vi "chr63204A_Mode_selector_Lowlevel.vi"(8 "error in (no error)":errorcluster, 10 "Mode":T1(ring), 11 "VISA resource name":refnum<visa-resource-name>) -> (0 "error out":errorcluster, 3 "VISA resource name out":refnum<visa-resource-name>)   [LabVIEW 2020]
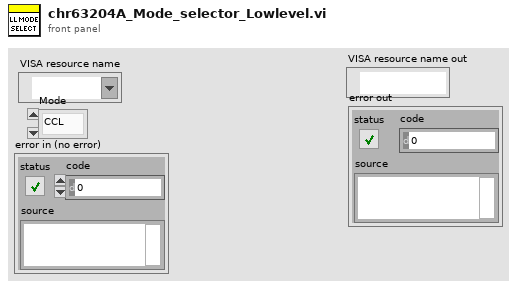
[diagram p1: front panel]
types:
  T1 = enum16{"CCL", "CCM", "CCH", "CRL", "CRM", "CRH", "CVL", "CVM", "CVH", "CPL", "CPM", "CPH", "CCDL", "CCDM", "CCDH", "CRDL", "CRDM", "CRDH", "BATL", "BATM", "BATH", "SWDL", "SWDM", "SWDH", "OCPL", "OCPM", "OCPH", "CCSL", "CCSM", "CCSH", "CZL", "CZM", "CZH", "CVCC", "CRCC", "CVCR", "AUTO", "PROG", "UDWL", "UDWM", "UDWH", "EXTL", "EXTM", "EXTH"}
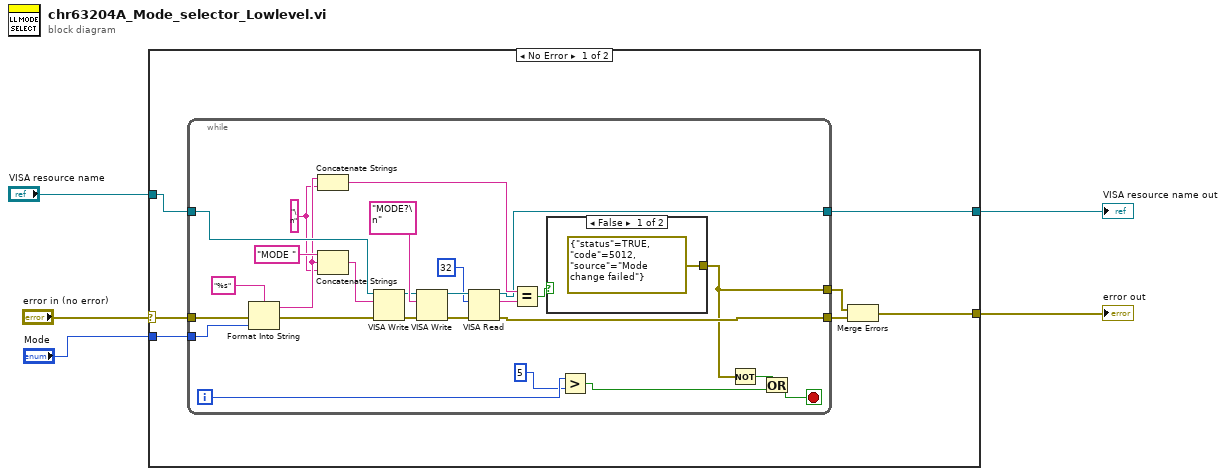
[diagram p0: block diagram]
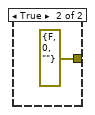
[diagram p2: hidden frame]
diagram:
  n1 = case shown="No Error" "error in (no error)" {
    selector: "error in (no error)" -> [w11 w41]
    tunnel: "VISA resource name" -> [w10 w42]
    tunnel: "Mode" -> [w12 _]
    tunnel: [w8 w42] -> w2
    tunnel: [w7 w41] -> w1
    frame No Error {
      n2 = while {
        tunnel: w12 -> [w38]
        tunnel: w11 -> [w36]
        tunnel: [w20] -> w9
        tunnel: w10 -> [w35]
        tunnel: [w19] -> w8
        tunnel: [w13] -> w6
        i -> [w18]
        stop <- w15 stop-if-true
        w24 = "\n" ("string")
        n3 = Format Into String(format string="%s", error in=w36, w38) -> (resulting string=w25:string, error out=w34:errorcluster)  [unwired: 1 in]
        n4 = Concatenate Strings(w25, w24) -> (w22:string)
        n5 = Concatenate Strings("MODE " ("string"), w25, w24) -> (w33:string)
        n6 = VISA Write(VISA resource name=w35, write buffer=w33, error in (no error)=w34) -> (VISA resource name out=w30:refnum<visa-resource-name>, error out=w29:errorcluster)  [unwired: 1 out]
        n7 = VISA Write(VISA resource name=w30, write buffer="MODE?\n", error in (no error)=w29) -> (VISA resource name out=w28:refnum<visa-resource-name>, error out=w27:errorcluster)  [unwired: 1 out]
        n8 = VISA Read(VISA resource name=w28, byte count=u32 32, error in (no error)=w27) -> (VISA resource name out=w19:refnum<visa-resource-name>, read buffer=w23:string, error out=w20:errorcluster)  [unwired: 1 out]
        n9 = Equal?(x=w22, y=w23) -> (x = y?=w21:bool)
        n10 = case shown="False" w21 {
          tunnel: [errorcluster {"status"=TRUE, "code"=5012, "source"="Mode change failed"} ("error constant") errorcluster {"status"=FALSE, "code"=0, "source"=""} ("error constant")] -> w13
          frame False {
          }
          frame True {
          }
        }
        n11 = Greater?(x=w18, y=5) -> (0:w16:bool)
        n12 = Not(x=w13) -> (.not. x?=w14:bool)
        n13 = Or(x=w14, y=w16) -> (x .or. y?=w15:bool)
      }
      n14 = Merge Errors(w6, w9) -> (w7:errorcluster)
    }
    frame Error {
    }
  }
  "VISA resource name out" <- w2
  "error out" <- w1
